vi "build_data_save_paths.vi"(4 "overwrite":bool, 6 "note-blob":string, 8 "base-file-name":string="cs-traj10-500.csv", 11 "data-root":path) -> (0 "output-meta-data-name":string, 1 "output-data-name":string, 2 "output-meta-data-path":path, 3 "output-data-path":path, 7 "input-data-path":path)   [LabVIEW 2017]
uses:
  <vilib>/regexp/Match Regular Expression.xnode
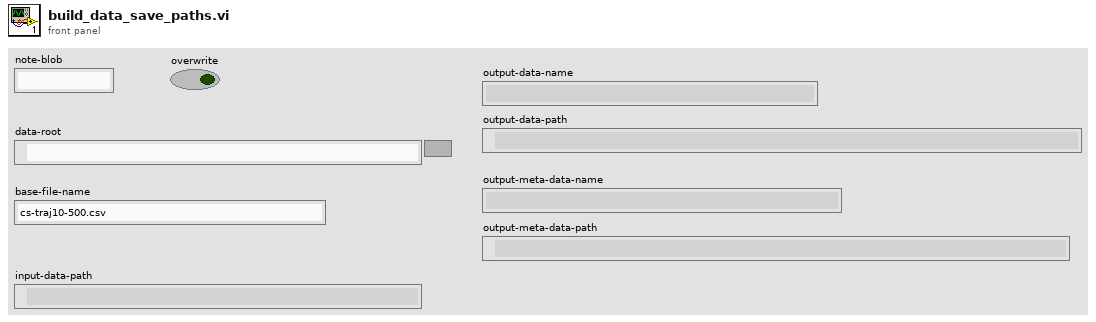
[diagram p1: front panel]
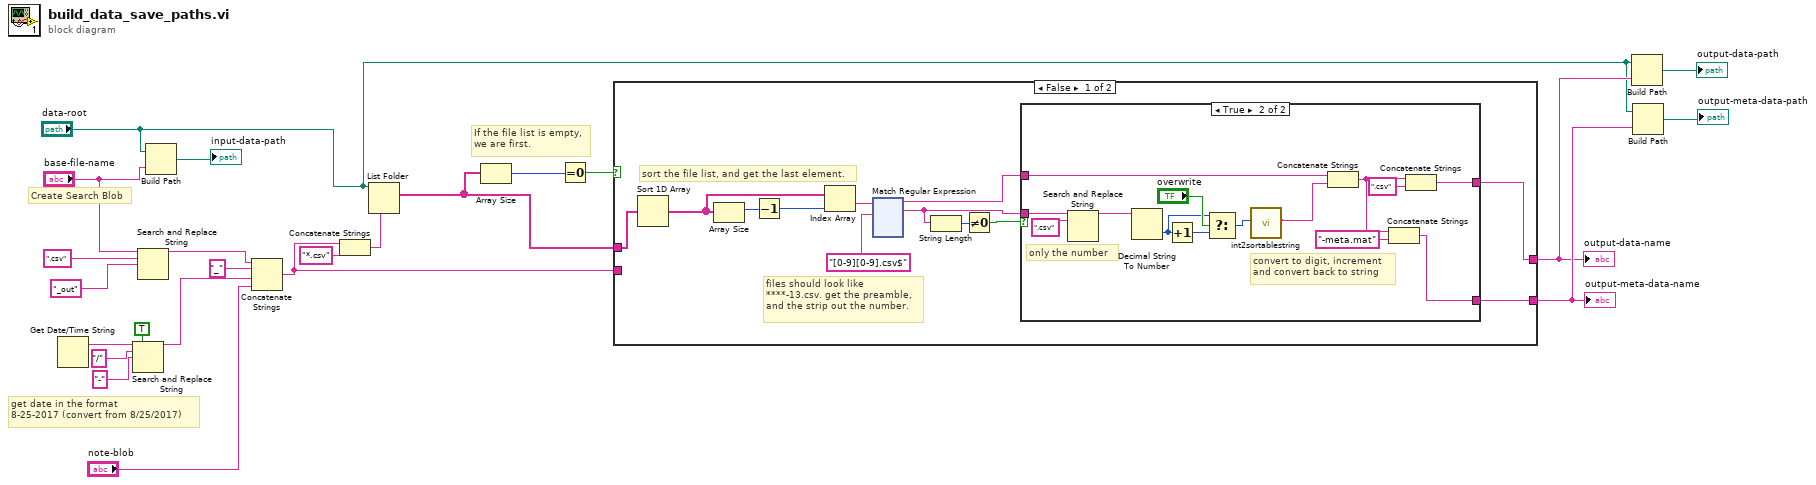
[diagram p0: block diagram]
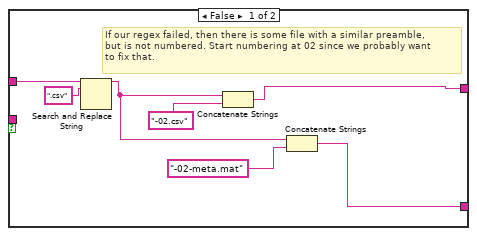
[diagram p2: hidden frame]
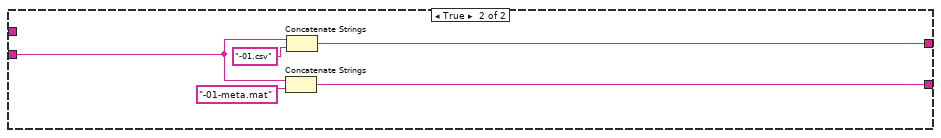
[diagram p3: hidden frame]
diagram:
  # "If the file list is empty,\nwe are first."
  # "Create Search Blob"
  # "get date in the format\n8-25-2017 (convert from 8/25/2017)"
  n1 = Get Date/Time String() -> (date string=w22:string)  [unwired: 3 in, 1 out]
  n2 = Search and Replace String(replace all?=TRUE ("replace all? (F)"), input string=w22, search string="/", replace string="-") -> (result string=w18:string)  [unwired: 4 in, 3 out]
  n3 = Search and Replace String(input string="base-file-name", search string=".csv", replace string="_out" ("replace string (\"\")")) -> (result string=w17:string)  [unwired: 5 in, 3 out]
  n4 = Build Path(base path="data-root", name or relative path="base-file-name") -> (appended path=→"input-data-path":path)
  n5 = Concatenate Strings(w17, "_", w18, "note-blob") -> (w10:string)
  n6 = Concatenate Strings(w10, "*.csv") -> (w11:string)
  n7 = List Folder(path="data-root", pattern=w11) -> (filenames=w9:string[])  [unwired: 2 in, 3 out]
  n8 = Array Size(array=w9) -> (size(s)=w14:i32)
  n9 = Equal To 0?(x=w14) -> (x = 0?=w13:bool)
  n10 = case shown="False" w13 {
    tunnel: w10 -> [_ w171]
    tunnel: [w29 w173] -> w5
    tunnel: [w28 w172] -> w6
    tunnel: w9 -> [w35 _]
    frame False {
      # "files should look like\n****-13.csv. get the preamble,\nand the strip out the number."
      # "sort the file list, and get the last element."
      n11 = Sort 1D Array(array=w35) -> (sorted array=w30:string[])
      n12 = Array Size(array=w30) -> (size(s)=w32:i32)
      n13 = Decrement(x=w32) -> (x-1=w31:i32)
      n14 = Index Array(array=w30, index=w31) -> (element=w34:string)
      n15 = xnode "Match Regular Expression"("input string"=w34, "regular expression"="[0-9][0-9].csv$") -> ("before match"=w27:string, "whole match"=w26:string)  [unwired: 4 in, 3 out]
      n16 = String Length(string=w26) -> (length=w25:i32)
      n17 = Not Equal To 0?(x=w25) -> (x != 0?=w24:bool)
      n18 = case shown="True" w24 {
        tunnel: w26 -> [_ w56]
        tunnel: [w40 w50] -> w29
        tunnel: [w41 w49] -> w28
        tunnel: w27 -> [w37 w48]
        frame False {
          # "If our regex failed, then there is some file with a similar preamble,\nbut is not numbered. Start numbering at 02 since we probably want\nto fix that."
          n19 = Search and Replace String(input string=w37, search string=".csv") -> (result string=w36:string)  [unwired: 6 in, 3 out]
          n20 = Concatenate Strings(w36, "-02.csv" ("string")) -> (w40:string)
          n21 = Concatenate Strings(w36, "-02-meta.mat" ("string")) -> (w41:string)
        }
        frame True {
          # "convert to digit, increment\nand convert back to string"
          # "only the number"
          n22 = Search and Replace String(input string=w56, search string=".csv") -> (result string=w54:string)  [unwired: 6 in, 3 out]
          n23 = Decimal String To Number(string=w54) -> (number=w43:i32)  [unwired: 2 in, 1 out]
          n24 = Increment(x=w43) -> (x+1=w46:i32)
          n25 = Select(t=w43, s="overwrite", f=w46) -> (s? t:f=w45:i32)
          n26 = call "int2sortablestring.vi"("int"=w45) -> ("tens-sortable-string"=w47:string)  [unwired: 10 in]
          n27 = Concatenate Strings(w48, w47) -> (w53:string)
          n28 = Concatenate Strings(w53, "-meta.mat" ("string")) -> (w49:string)
          n29 = Concatenate Strings(w53, ".csv" ("string")) -> (w50:string)
        }
      }
    }
    frame True {
      n30 = Concatenate Strings(w171, "-01-meta.mat") -> (w172:string)
      n31 = Concatenate Strings(w171, "-01.csv") -> (w173:string)
    }
  }
  "output-data-name" <- w5
  "output-meta-data-name" <- w6
  n32 = Build Path(base path="data-root", name or relative path=w5) -> (appended path=→"output-data-path":path)
  n33 = Build Path(base path="data-root", name or relative path=w6) -> (appended path=→"output-meta-data-path":path)
